vi "Relative Accuracy Ae.vi"(0 "VISA resource name":refnum<visa-resource-name>, 1 "Temperature (5 C)":dbl=5.0 min=5.0 max=45.0 format="%.2f", 2 "Ka":dbl format="%^.2e", 3 "Kb":dbl format="%^.2e", 4 "Kc":dbl format="%.3f", 5 "error in (no error)":errorcluster, 6 "Kaa":dbl format="%.3f", 7 "Kd":dbl format="%^.2e", 8 "Kbb":dbl format="%^.2e", 9 "Dx":dbl format="%.3f", 10 "A":dbl format="%.3f", 11 "Qx":dbl format="%.3f", 12 "Meas. Type (0:Z,Y)":enum16{"Z,Y", "L C X B", "R G"}(ring)) -> (14 "VISA resource name out":refnum<visa-resource-name>, 16 "Ae Accuracy":dbl format="%.2f", 19 "error out":errorcluster)   [LabVIEW 2015, in "Agilent 428X Series.lvlib"]
doc: "This Vi returns the value of relative accuracy parameter Ae.\nAe is given as:\nAe=(A+(Ke+Kaa+Kb*Kbb+Kc)*100+Kd)*Ke\n\nDisclaimer: All accuracy calculation VI's are not part of the original \n driver. They are provided for supplementry purpose only.\n If user desires very high accuracy data, please do or \n check the calculation seperately."
uses:
  <instrlib>/Agilent 428X Series/Agilent 428X Series.lvlib
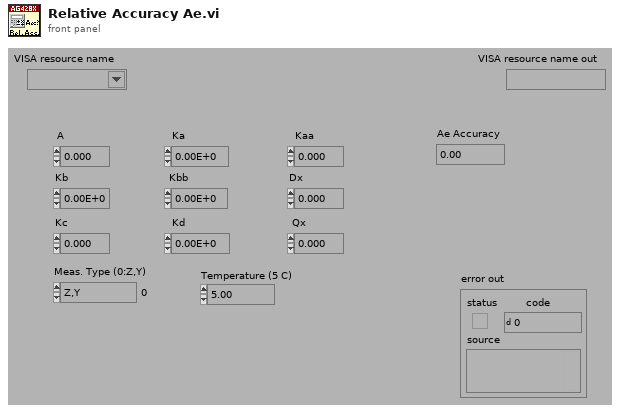
[diagram p1: front panel]
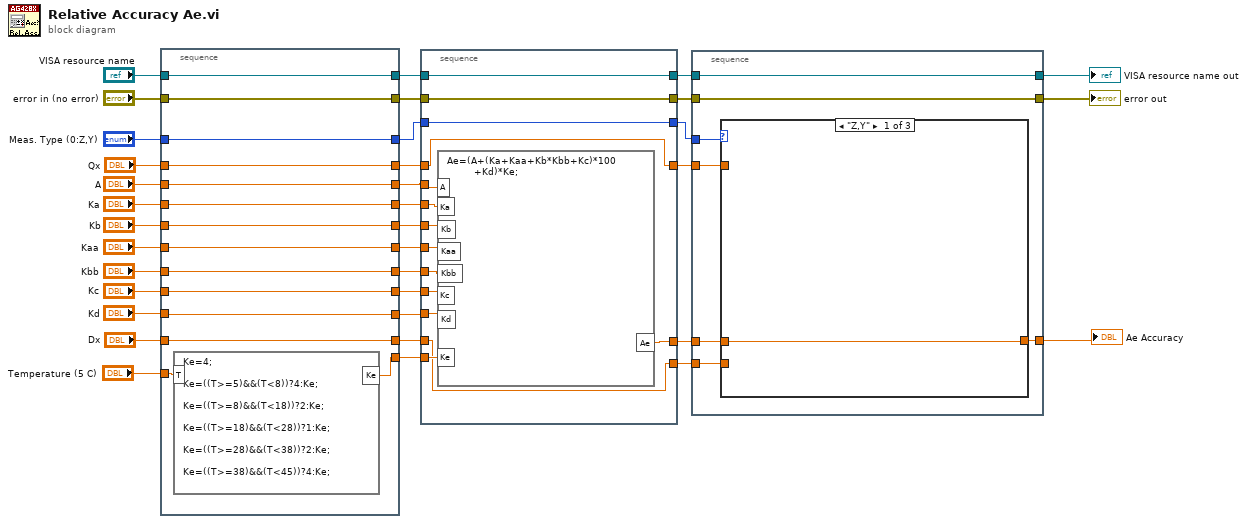
[diagram p0: block diagram]
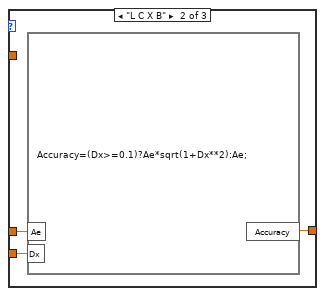
[diagram p2: hidden frame]
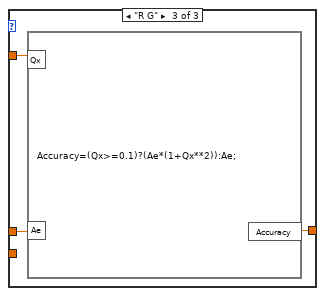
[diagram p3: hidden frame]
diagram:
  n1 = stacked-sequence {
    tunnel: "Temperature (5 C)" -> [w49]
    tunnel: "VISA resource name" -> [w48]
    tunnel: "error in (no error)" -> [w47]
    tunnel: [w48] -> w32
    tunnel: [w47] -> w31
    tunnel: "Dx" -> [w41]
    tunnel: "Qx" -> [w44]
    tunnel: "A" -> [w45]
    tunnel: "Ka" -> [w46]
    tunnel: [w46] -> w20
    tunnel: [w45] -> w19
    tunnel: [w44] -> w18
    tunnel: "Meas. Type (0:Z,Y)" -> [w43]
    tunnel: [w43] -> w15
    tunnel: [w42] -> w13
    tunnel: [w41] -> w12
    tunnel: "Kb" -> [w40]
    tunnel: [w40] -> w9
    tunnel: "Kaa" -> [w39]
    tunnel: [w39] -> w7
    tunnel: "Kbb" -> [w38]
    tunnel: [w38] -> w5
    tunnel: "Kc" -> [w37]
    tunnel: [w37] -> w3
    tunnel: "Kd" -> [w36]
    tunnel: [w36] -> w1
    frame #0 {
      n2 = formula code="Ke=4;\n\nKe=((T>=5)&&(T<8))?4:Ke;\n\nKe=((T>=8)&&(T<18))?2:Ke;\n\nKe=((T>=18)&&(T<28))?1:Ke;\n\nKe=((T>=28)&&(T<38))?2:Ke;\n\nKe=((T>=38)&&(T<45))?4:Ke;"("T"=w49) -> ("Ke"=w42:dbl)
    }
  }
  n3 = stacked-sequence {
    tunnel: w32 -> [w62]
    tunnel: w31 -> [w63]
    tunnel: [w62] -> w28
    tunnel: [w63] -> w27
    tunnel: [w61] -> w30
    tunnel: w1 -> [w60]
    tunnel: w3 -> [w59]
    tunnel: w5 -> [w58]
    tunnel: w7 -> [w57]
    tunnel: w9 -> [w56]
    tunnel: w20 -> [w55]
    tunnel: w19 -> [w54]
    tunnel: w18 -> [w53]
    tunnel: [w53] -> w17
    tunnel: w15 -> [w52]
    tunnel: [w52] -> w14
    tunnel: w13 -> [w51]
    tunnel: w12 -> [w50]
    tunnel: [w50] -> w11
    frame #0 {
      n4 = formula code="Ae=(A+(Ka+Kaa+Kb*Kbb+Kc)*100\n         +Kd)*Ke;"("Ke"=w51, "Kd"=w60, "Kc"=w59, "A"=w54, "Kb"=w56, "Ka"=w55, "Kaa"=w57, "Kbb"=w58) -> ("Ae"=w61:dbl)
    }
  }
  n5 = stacked-sequence {
    tunnel: w17 -> [w70]
    tunnel: w30 -> [w69]
    tunnel: [w68] -> w29
    tunnel: w27 -> [w67]
    tunnel: [w67] -> w26
    tunnel: w28 -> [w66]
    tunnel: [w66] -> w25
    tunnel: w14 -> [w65]
    tunnel: w11 -> [w64]
    frame #0 {
      n6 = case shown="\"Z,Y\"" w65 {
        tunnel: [w71 w74 w77] -> w68
        tunnel: w69 -> [w71 w73 w76]
        tunnel: w70 -> [_ _ w75]
        tunnel: w64 -> [_ w72 _]
        frame "Z,Y" {
        }
        frame "L C X B" {
          n7 = formula code="Accuracy=(Dx>=0.1)?Ae*sqrt(1+Dx**2):Ae;"("Dx"=w72, "Ae"=w73) -> ("Accuracy"=w74:dbl)
        }
        frame "R G" {
          n8 = formula code="Accuracy=(Qx>=0.1)?(Ae*(1+Qx**2)):Ae;"("Qx"=w75, "Ae"=w76) -> ("Accuracy"=w77:dbl)
        }
      }
    }
  }
  "VISA resource name out" <- w25
  "error out" <- w26
  "Ae Accuracy" <- w29
